vi "Boolean Counter 1.vi"() -> ()   [LabVIEW 2020]
panel:
  out "Numeric":i32
  out "x":dbl
  out "x+y":dbl
  in  "stop":bool
  in  "Boolean":bool
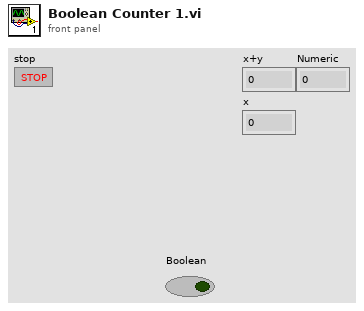
[diagram p1: front panel]
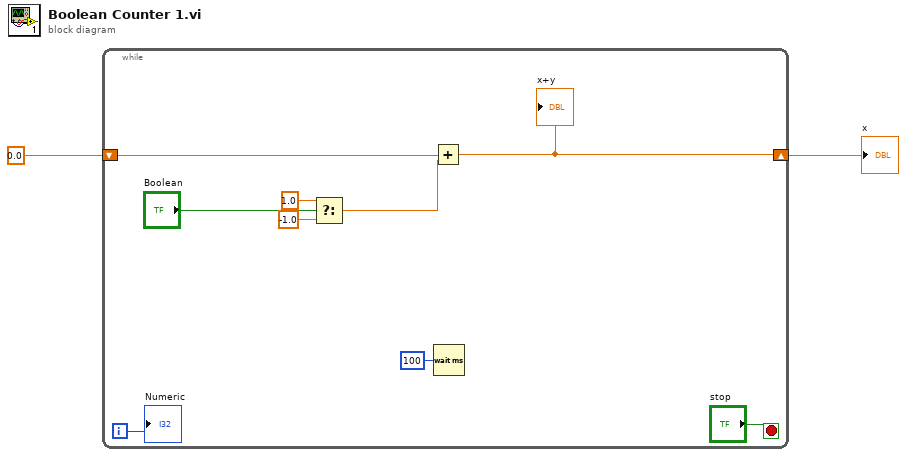
[diagram p0: block diagram]
diagram:
  n1 = while {
    shift-right: [w10] -> w1
    shift-left: 0.0 ("x") -> [w11]
    i -> [w3]
    stop <- "stop" stop-if-true
    n2 = Select(t=1.0, s="Boolean", f=-1.0) -> (s? t:f=w8:dbl)
    n3 = Add(x=w11, y=w8) -> (x+y=w10:dbl)
    "x+y" <- w10
    n4 = Wait (ms)(milliseconds to wait=u32 100) -> ()  [unwired: 1 out]
    "Numeric" <- w3
  }
  "x" <- w1
